vi "Translate WAV file.vi"(8 "Settings":T1={"Name of test"="ScratchPad", "Date"=timestamp(0 s since 1904-01-01), "Location"="Home", "Template"="ScratchPad", "Soundcard"="OCTA-CAPTURE", "resolution"=32, "Sampling rate"=48000, "Ch1 Gain "=25.0, "Ch2 Gain"=10.0, "Sample time (s)"=0.3, "Pre-trigger (s)"=0.001, "Hammer Threshold"=0.021311, "Positions"=12, "Taps/Position"=5, "Set Names"="H,V", "Freq resolution"=1.0, "Hammer cutoff"=0.025, "Mic cutoff"=0.25, "Double bounce "=0.01, "Hammer Cal"=1.0, "dB Offset"=0.0, "Accel Cal"=10.0, "Vibrometer Cal"=1.0, "Mic Cal"=1.0, "Output"=2, "Voltage Cal"=1.0, "Vibrometer Port"="ASRL27::INSTR", "Range"=4, "High Pass"=2, "Bandwidth"=4, "X Range"=[{"Minimum"=200.0, "Maximum"=10000.0, "Increment"=10.0, "Minor Increment"=100.0, "Start"=200.0}, {"Minimum"=0.0, "Maximum"=0.05, "Increment"=0.025, "Minor Increment"=0.0025, "Start"=0.0}, {"Minimum"=0.0, "Maximum"=0.3, "Increment"=0.1, "Minor Increment"=0.01, "Start"=0.0}, {"Minimum"=200.0, "Maximum"=10000.0, "Increment"=10.0, "Minor Increment"=100.0, "Start"=1000.0}], "Y Range"=[{"Minimum"=-25.0, "Maximum"=0.0, "Increment"=5.0, "Minor Increment"=1.0, "Start"=-25.0}, {"Minimum"=-0.1, "Maximum"=0.1, "Increment"=0.05, "Minor Increment"=0.01, "Start"=-0.1}, {"Minimum"=-0.1, "Maximum"=0.1, "Increment"=0.05, "Minor Increment"=0.01, "Start"=-0.1}, {"Minimum"=-20.0, "Maximum"=20.0, "Increment"=2.0, "Minor Increment"=0.5, "Start"=-20.0}], "dB Spread"=40.0, "Trigger"=0, "Ch_1"=1, "Ch_2"=2, "flip?"=FALSE, "60Hz"=FALSE, "Time offset"=0.0, "Piezo Cal"=1.0, "Default Notes"=""} {"Ch_2" min=1 step=1; "Ch_1" min=1 max=100 step=1; "Trigger" items=["Hammer (force)", "Self-tap", "Spacebar"]; "Bandwidth" items=["1 kHz"=1, "5 kHz"=5, "10 kHz"=10, "25 kHz"=25, "50 kHz"=50, "100 kHz"=100]; "High Pass" items=["Off", "13 Hz", "104 Hz"]; "Range" items=["10 mm/s"=1, "20 mm/s"=2, "50 mm/s"=5, "100 mm/s"=10, "200 mm/s"=20, "500 mm/s"=50, "1 m/s"=100, "2 m/s"=200]; "Output" items=["Accelerometer", "Speed (from acceleration)", "Microphone", "Vibrometer", "Piezo"]; "Voltage Cal" format="%#_13g"; "Ch2 Gain" format="%#_13g"; "Ch1 Gain" format="%#_13g"; "Double bounce" min=0.0; "Mic cutoff" min=0.0 format="%#_4g"; "Hammer cutoff" min=0.0 format="%#_4g"; "Freq resolution" min=0.0; "Pre-trigger (s)" format="%#_13g"; "Date" format="%<%H:%M\n%d/%m/%y>T"; "resolution" items=["16 bit"=16, "24 bit"=24, "32 bit"=32]; "Sampling rate" items=["22050 samp/s"=22050, "44100 samp/s"=44100, "48000 samp/s"=48000]}, 10 "Name of test":string, 11 "appended path":path) -> (0 "Settings Out":T1={"Name of test"="", "Date"=timestamp(0 s since 1904-01-01), "Location"="", "Template"="", "Soundcard"="", "resolution"=32, "Sampling rate"=48000, "Ch1 Gain "=25.0, "Ch2 Gain"=10.0, "Sample time (s)"=0.3, "Pre-trigger (s)"=0.01, "Hammer Threshold"=10.0, "Positions"=12, "Taps/Position"=5, "Set Names"="", "Freq resolution"=10.0, "Hammer cutoff"=0.0, "Mic cutoff"=0.0, "Double bounce "=0.0, "Hammer Cal"=1.0, "dB Offset"=0.0, "Accel Cal"=1.0, "Vibrometer Cal"=1.0, "Mic Cal"=1.0, "Output"=2, "Voltage Cal"=1.0, "Vibrometer Port"="ASRL27::INSTR", "Range"=50, "High Pass"=2, "Bandwidth"=25, "X Range"=[], "Y Range"=[], "dB Spread"=0.0, "Trigger"=0, "Ch_1"=1, "Ch_2"=2, "flip?"=FALSE, "60Hz"=FALSE, "Time offset"=0.0, "Piezo Cal"=1.0, "Default Notes"=""} {"Ch_2" min=1 step=1; "Ch_1" min=1 max=100 step=1; "Trigger" items=["Hammer (force)", "Self-tap", "Spacebar"]; "Bandwidth" items=["1 kHz"=1, "5 kHz"=5, "10 kHz"=10, "25 kHz"=25, "50 kHz"=50, "100 kHz"=100]; "High Pass" items=["Off", "13 Hz", "104 Hz"]; "Range" items=["10 mm/s"=1, "20 mm/s"=2, "50 mm/s"=5, "100 mm/s"=10, "200 mm/s"=20, "500 mm/s"=50, "1 m/s"=100, "2 m/s"=200]; "Output" items=["Accelerometer", "Speed (from acceleration)", "Microphone", "Vibrometer", "Piezo"]; "Voltage Cal" format="%#_13g"; "Ch2 Gain" format="%#_13g"; "Ch1 Gain" format="%#_13g"; "Double bounce" min=0.0; "Mic cutoff" min=0.0 format="%#_4g"; "Hammer cutoff" min=0.0 format="%#_4g"; "Freq resolution" min=0.0; "Pre-trigger (s)" format="%#_13g"; "Date" format="%<%H:%M\n%d/%m/%y>T"; "resolution" items=["16 bit"=16, "24 bit"=24, "32 bit"=32]; "Sampling rate" items=["22050 samp/s"=22050, "44100 samp/s"=44100, "48000 samp/s"=48000]}, 1 "data":T2={"Hammer"=[], "Hammer Spectra"=[{1.0, "df"=1.0, "FFT {X}"=array[24000 elements]}], "Microphone"=[{0.0, "dt"=2.0833333333333333e-05, "Y"=array[14400 elements]}], "Microphone Spectra"=[{"x0"=1.0, "df"=1.0, array[24000 elements]}], "Average FRF"=[{1.0, "df"=1.0, array[24000 elements]}, {1.0, "df"=1.0, array[24000 elements]}]}, 2 "data 2":waveform(dbl)[](graph), 3 "Average FRF out":cluster{"x0":dbl, "df":dbl, dbl[]}, 4 "data":waveform(dbl)[](graph), 5 "Complex FRF":cluster{dbl, "df":dbl, cdb[]}, 6 "# pts":i32)   [LabVIEW 2022 SP3]
uses:
  PreferencesControl.ctl
panel:
  out "Array":waveform(dbl)[](array[waveform])
  # "Hz"
  # "dB"
  # "dB"
  # "sec"
  # "sec"
  # "mV/Pa"
  # "mV/m/s2"
  # "mV/mm/s"
  # "V/N"
  # "sec"
  # "sec"
  # "mV/N"
  # "a.u."
  # "a.u."
  # "sec"
  # "Hz"
  # "dB"
  # "dB"
  # "sec"
  # "sec"
  # "mV/Pa"
  # "mV/m/s2"
  # "mV/mm/s"
  # "V/N"
  # "sec"
  # "sec"
  # "mV/N"
  # "a.u."
  # "a.u."
  # "sec"
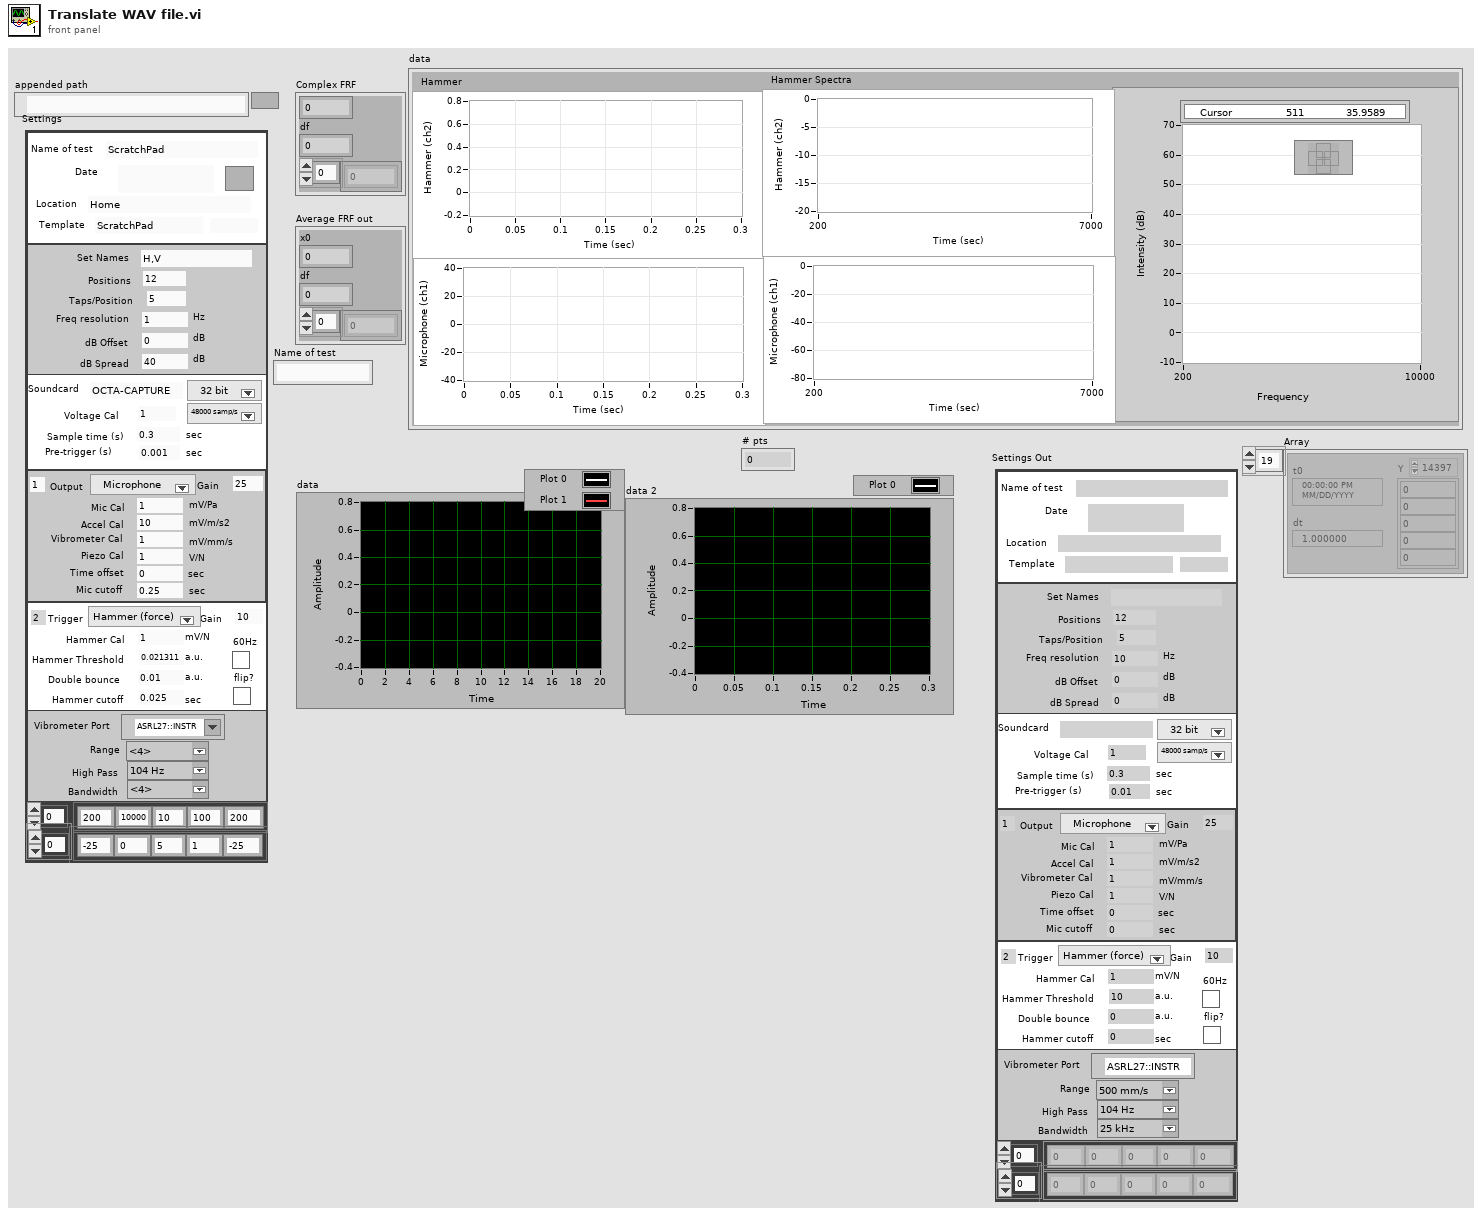
[diagram p1: front panel]
types:
  T1 = typedef "PreferencesControl.ctl" = cluster{"Name of test":string, "Date":timestamp, "Location":string, "Template":string, "Soundcard":string, "resolution":u16, "Sampling rate":u16, "Ch1 Gain ":dbl, "Ch2 Gain":dbl, "Sample time (s)":dbl, "Pre-trigger (s)":dbl, "Hammer Threshold":dbl, "Positions":i16, "Taps/Position":i16, "Set Names":string, "Freq resolution":dbl, "Hammer cutoff":dbl, "Mic cutoff":dbl, "Double bounce ":dbl, "Hammer Cal":dbl, "dB Offset":dbl, "Accel Cal":dbl, "Vibrometer Cal":dbl, "Mic Cal":dbl, "Output":u16, "Voltage Cal":dbl, "Vibrometer Port":refnum<visa-resource-name>, "Range":u16, "High Pass":u16, "Bandwidth":u16, "X Range":cluster{"Minimum":dbl, "Maximum":dbl, "Increment":dbl, "Minor Increment":dbl, "Start":dbl}[], "Y Range":cluster{"Minimum":dbl, "Maximum":dbl, "Increment":dbl, "Minor Increment":dbl, "Start":dbl}[], "dB Spread":dbl, "Trigger":u16, "Ch_1":u8, "Ch_2":u8, "flip?":bool, "60Hz":bool, "Time offset":dbl, "Piezo Cal":dbl, "Default Notes":string}
  T2 = cluster{"Hammer":cluster{dbl, "dt":dbl, "Y":dbl[]}[], "Hammer Spectra":cluster{dbl, "df":dbl, "FFT {X}":dbl[]}[], "Microphone":cluster{dbl, "dt":dbl, "Y":dbl[]}[], "Microphone Spectra":cluster{"x0":dbl, "df":dbl, dbl[]}[], "Average FRF":cluster{dbl, "df":dbl, dbl[]}[]}
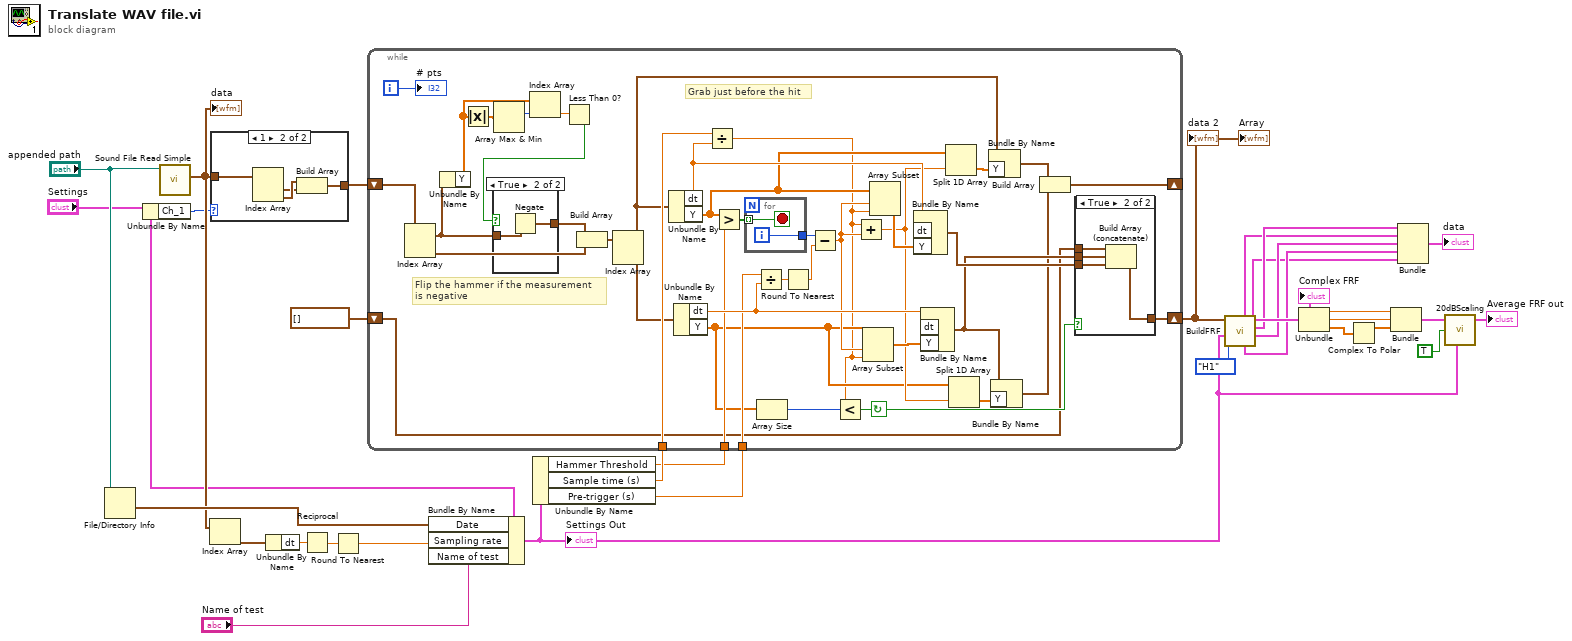
[diagram p0: block diagram]
diagram:
  n1 = File/Directory Info(path="appended path") -> (last mod=w23:timestamp)  [unwired: 1 in, 6 out]
  n2 = Unbundle By Name("Settings") -> ("Ch_1"=w9:u8)
  n3 = call <vilib>:"Sound File Read Simple.vi"("path"="appended path") -> ("data"=w22:waveform(dbl)[])  [unwired: 7 in, 3 out]
  "data" <- w22
  n4 = Index Array(array=w22) -> (element=w21:waveform(dbl))  [unwired: 1 in]
  n5 = case shown="1" w9 {
    tunnel: w22 -> [w33 w37]
    tunnel: [w33 w34] -> w32
    frame 0, Default {
    }
    frame 1 {
      n6 = Index Array(array=w37) -> (element #1=w35:waveform(dbl), element #2=w36:waveform(dbl))  [unwired: 2 in]
      n7 = Build Array(w36, w35) -> (w34:waveform(dbl)[])
    }
  }
  n8 = Unbundle By Name(w21) -> ("dt"=w20:dbl)
  n9 = Reciprocal(x=w20) -> (1/x=w19:dbl)
  n10 = Round To Nearest(number=w19) -> (nearest integer value=w18:dbl)
  n11 = Bundle By Name(cluster="Settings", "Date"=w23, "Sampling rate"=w18, "Name of test"="Name of test") -> (w8:T1)
  "Settings Out" <- w8
  n12 = Unbundle By Name(w8) -> ("Hammer Threshold"=w5:dbl, "Sample time (s)"=w17:dbl, "Pre-trigger (s)"=w4:dbl)
  n13 = while {
    tunnel: w17 -> [w72]
    tunnel: w5 -> [w57]
    tunnel: w4 -> [w56]
    shift-right: [w46] -> _
    shift-left: w32 -> [w77]
    shift-right: [w45] -> w3
    shift-left: waveform(dbl)[] [] -> [w38]
    i -> [w40]
    stop <- w41 continue-if-true
    # "Grab just before the hit"
    # "Flip the hammer if the measurement\nis negative"
    n14 = Index Array(array=w77) -> (element #1=w65:waveform(dbl), element #2=w67:waveform(dbl))  [unwired: 2 in]
    n15 = Unbundle By Name(w65) -> ("Y"=w63:dbl[])
    n16 = Absolute Value(x=w63) -> (abs(x)=w64:dbl[])
    n17 = Array Max & Min(array=w64) -> (max index (indices)=w62:i32)  [unwired: 3 out]
    n18 = Index Array(array=w63, index=w62) -> (element=w61:dbl)
    n19 = Less Than 0?(x=w61) -> (x < 0?=w60:bool)
    n20 = case shown="True" w60 {
      tunnel: [w83 w85] -> w66
      tunnel: w65 -> [w83 w84]
      frame False {
      }
      frame True {
        n21 = Negate(x=w84) -> (-x=w85:waveform(dbl))
      }
    }
    n22 = Build Array(w66, w67) -> (w73:waveform(dbl)[])
    n23 = Index Array(array=w73) -> (element #1=w52:waveform(dbl), element #2=w58:waveform(dbl))  [unwired: 2 in]
    n24 = Unbundle By Name(w52) -> ("dt"=w75:dbl, "Y"=w55:dbl[])
    n25 = Unbundle By Name(w58) -> ("dt"=w70:dbl, "Y"=w43:dbl[])
    n26 = Divide(x=w72, y=w75) -> (x/y=w39:dbl)
    n27 = Greater?(x=w55, y=w57) -> (0:w76:bool[])
    n28 = for {
      tunnel: w76 -> [w87] mode=indexing
      tunnel: [w86] -> w44
      i -> [w86]
      stop <- w87 stop-if-true
    }
    n29 = Divide(x=w56, y=w70) -> (x/y=w69:dbl)
    n30 = Array Size(array=w43) -> (size(s)=w42:i32)
    n31 = Round To Nearest(number=w69) -> (nearest integer value=w68:dbl)
    n32 = Subtract(x=w44, y=w68) -> (x-y=w54:dbl)
    n33 = Less?(x=w39, y=w42) -> (x < y?=w41:bool)
    n34 = Add(x=w39, y=w54) -> (x+y=w51:dbl)
    n35 = Array Subset(array=w43, index=w54, length=w39) -> (w74:dbl[])
    n36 = Array Subset(array=w55, index=w54, length=w39) -> (w59:dbl[])
    n37 = Bundle By Name("dt"=w75, "Y"=w59) -> (w71:waveform(dbl))  [unwired: 1 in]
    n38 = Bundle By Name("dt"=w70, "Y"=w74) -> (w49:waveform(dbl))  [unwired: 1 in]
    n39 = Split 1D Array(array=w55, index=w51) -> (second subarray=w53:dbl[])  [unwired: 1 out]
    n40 = Split 1D Array(array=w43, index=w51) -> (second subarray=w50:dbl[])  [unwired: 1 out]
    n41 = Bundle By Name(cluster=w52, "Y"=w53) -> (w48:waveform(dbl))
    n42 = Bundle By Name(cluster=w49, "Y"=w50) -> (w47:waveform(dbl))
    n43 = Build Array(w48, w47) -> (w46:waveform(dbl)[])
    n44 = case shown="True" w41 {
      tunnel: w71 -> [_ w82]
      tunnel: w49 -> [_ w81]
      tunnel: [w78 w80] -> w45
      tunnel: w38 -> [w78 w79]
      frame False {
      }
      frame True {
        n45 = Build Array (concatenate)(w79, w81, w82) -> (w80:waveform(dbl)[])
      }
    }
    "# pts" <- w40
  }
  "data 2" <- w3
  "Array" <- w3
  n46 = call "BuildFRF.vi"("Method"=enum16{"Sqrt(H1H2)", "H1", "H2"}."H1", "Settings"=w8, "Data In"=w3) -> ("Average FRF"=w12:cluster{dbl, "df":dbl, dbl[]}[], "Microphone"=w14:cluster{dbl, "dt":dbl, "Y":dbl[]}[], "Hammer"=w16:cluster{dbl, "dt":dbl, "Y":dbl[]}[], "Complex FRF"=w30:cluster{"t0":dbl, "dt":dbl, "Y":cdb[]}, "Microphone Spectra"=w13:cluster{"x0":dbl, "df":dbl, dbl[]}[], "Hammer Spectra"=w15:cluster{dbl, "df":dbl, "FFT {X}":dbl[]}[])  [unwired: 3 in]
  "Complex FRF" <- w30
  n47 = Unbundle(w30) -> ("t0"=w28:dbl, "dt"=w29:dbl, "Y"=w26:cdb[])
  n48 = Complex To Polar(r * e^(i*theta)=w26) -> (r=w27:dbl[])  [unwired: 1 out]
  n49 = Bundle("t0"=w28, "dt"=w29, w27) -> (w6:cluster{"t0":dbl, "dt":dbl, dbl[]})  [unwired: 1 in]
  n50 = Bundle("Hammer"=w16, "Hammer Spectra"=w15, "Microphone"=w14, "Microphone Spectra"=w13, "Average FRF"=w12) -> (→"data":T2)  [unwired: 1 in]
  n51 = call "20dBScaling.vi"("Average FRF in"=w6, "dB?"=TRUE, "Settings"=w8) -> ("Average FRF out"=→"Average FRF out":cluster{"x0":dbl, "df":dbl, dbl[]})  [unwired: 3 in, 1 out]
